vi "Global Cancel Control.vi"() -> ()   [LabVIEW 2024]
uses:
  Globals and TypeDefs/Type Definitions.llb/3 way Status.ctl
  Globals and TypeDefs/Global Varibal Control.vi
  Globals and TypeDefs/gStatus.vi
panel:
  out "Current Experiment Status":T2 {"Saving" items=["N.A.", "OK", "Busy", "Done"]; "Plotting" items=["N.A.", "OK", "Busy", "Done"]; "Buffer" items=["N.A.", "OK", "Busy", "Done"]; "Exposure" items=["N.A.", "OK", "Busy", "Done"]; "Spectrometer" items=["N.A.", "OK", "Busy", "Done"]; "Temperature" items=["N.A.", "OK", "Busy", "Done"]; "Field" items=["N.A.", "OK", "Busy", "Done"]}
  in  "Resume":bool
  in  "Cancel":bool
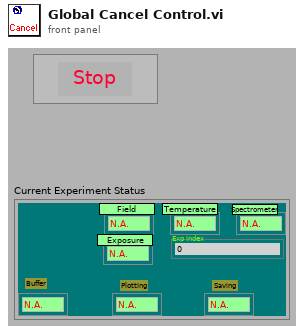
[diagram p1: front panel]
types:
  T1 = typedef "3 way Status.ctl" = u8
  T2 = cluster{"Exp Index":u32, "Field":T1, "Temperature":T1, "Spectrometer":T1, "Exposure":T1, "Buffer":T1, "Plotting":T1, "Saving":T1}
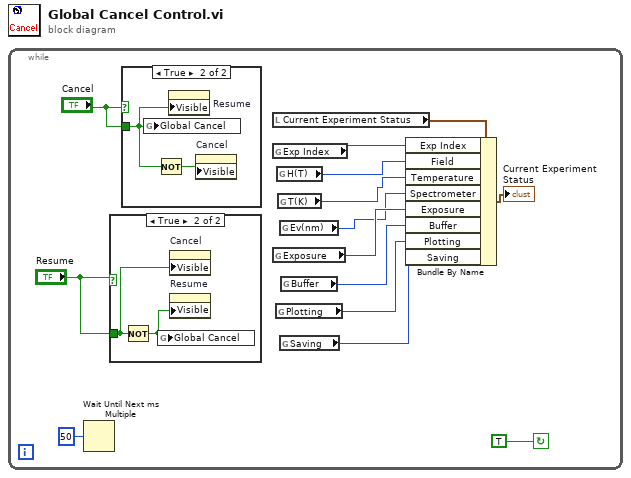
[diagram p0: block diagram]
diagram:
  n1 = while {
    stop <- TRUE continue-if-true
    n2 = Wait Until Next ms Multiple(millisecond multiple=u32 50) -> ()  [unwired: 1 out]
    n3 = case shown="True" "Resume" {
      tunnel: "Resume" -> [_ w16]
      frame False {
      }
      frame True {
        n4 = Not(x=w16) -> (.not. x?=w15:bool)
        n5 = global write "Global Varibal Control.vi" "Global Cancel"(w15) -> ()
        n6 = property on="Cancel" class="Bool"("Visible"=w16) -> ()  [unwired: 2 in, 2 out]
        n7 = property on="Resume" class="Bool"("Visible"=w15) -> ()  [unwired: 2 in, 2 out]
      }
    }
    n8 = case shown="True" "Cancel" {
      tunnel: "Cancel" -> [_ w17]
      frame False {
      }
      frame True {
        n9 = global write "Global Varibal Control.vi" "Global Cancel"(w17) -> ()
        n10 = Not(x=w17) -> (.not. x?=w18:bool)
        n11 = property on="Resume" class="Bool"("Visible"=w17) -> ()  [unwired: 2 in, 2 out]
        n12 = property on="Cancel" class="Bool"("Visible"=w18) -> ()  [unwired: 2 in, 2 out]
      }
    }
    n13 = local read "Current Experiment Status"() -> (w9:T2)
    n14 = global read "gStatus.vi" "Exp Index"() -> (w7:u32)
    n15 = global read "gStatus.vi" "Exposure"() -> (w8:T1)
    n16 = global read "gStatus.vi" "Plotting"() -> (w2:T1)
    n17 = global read "gStatus.vi" "H(T)"() -> (w6:T1)
    n18 = global read "gStatus.vi" "T(K)"() -> (w5:T1)
    n19 = global read "gStatus.vi" "Ev(nm)"() -> (w4:T1)
    n20 = global read "gStatus.vi" "Saving"() -> (w1:T1)
    n21 = global read "gStatus.vi" "Buffer"() -> (w3:T1)
    n22 = Bundle By Name(cluster=w9, "Exp Index"=w7, "Field"=w6, "Temperature"=w5, "Spectrometer"=w4, "Exposure"=w8, "Buffer"=w3, "Plotting"=w2, "Saving"=w1) -> (→"Current Experiment Status":T2)
  }
